vi "MainIdent RT.vi"() -> ()   [LabVIEW 2019]
doc: "The myRIO Project template acquires acceleration data from the onboard accelerometer and displays the changes of acceleration values in a waveform chart."
uses:
  CD1.ctl
  <vilib>/myRIO/Common/Instrument Driver Framework/myRIO v1.0/Encoder/typedefs/Encoder Signal Mode.ctl
  <vilib>/Platform/TimedLoop/XDataNode/timing_clust.ctl
  <vilib>/Platform/TimedLoop/XDataNode/nitl_modes.ctl
  <vilib>/Platform/TimedLoop/XDataNode/wakeup.ctl
  <vilib>/myRIO/Instrument Drivers/Onboard IO/PWM/typedefs/PWM Reference.ctl
  <vilib>/myRIO/Common/Instrument Driver Framework/Utilities/typedefs/myRIO Generic Hardware Reference.ctl
  <vilib>/myRIO/Common/Instrument Driver Framework/Utilities/typedefs/Hardware Version Enum.ctl
  <vilib>/myRIO/Common/Instrument Driver Framework/Utilities/typedefs/myRIO v1.0 Reference.ctl
  <vilib>/myRIO/Common/Instrument Driver Framework/Utilities/typedefs/Generic FPGA Reference.ctl
  <vilib>/myRIO/Common/Instrument Driver Framework/myRIO v1.0/PWM/typedefs/PWM Channels Enum.ctl
  <vilib>/myRIO/Instrument Drivers/Onboard IO/PWM/typedefs/PWM Configuration.ctl
  <vilib>/userDefined/High Color/nirio_resource_hc.ctl
  <vilib>/myRIO/Common/Instrument Driver Framework/myRIO v1.0/Encoder/typedefs/Encoder Configuration v1.0.ctl
  <vilib>/myRIO/Instrument Drivers/Onboard IO/Encoder/typedefs/Encoder Reference.ctl
  <vilib>/myRIO/Common/Instrument Driver Framework/myRIO v1.0/Encoder/typedefs/Encoder Channels Enum.ctl
  <vilib>/myRIO/Common/Instrument Driver Framework/myRIO v1.0/PWM/vis/myRIO v1.1 Open PWM.vi
  <vilib>/myRIO/Common/Instrument Driver Framework/myRIO v1.0/Encoder/vis/myRIO v1.1 Open Encoder.vi
  <vilib>/myRIO/Common/Instrument Driver Framework/Utilities/vis/Validate Channels.vi
  <vilib>/myRIO/Common/Instrument Driver Framework/myRIO v1.0/PWM/vis/myRIO v1.0 Reserve PWM.vi
  <vilib>/myRIO/Instrument Drivers/Onboard IO/PWM/vis/Set Duty Cycle and Frequency.vi
  <vilib>/myRIO/Common/Instrument Driver Framework/myRIO v1.0/Encoder/vis/myRIO v1.0 Reserve Encoder.vi
  <vilib>/myRIO/Common/Instrument Driver Framework/myRIO v1.0/Encoder/vis/myRIO v1.0 Close Encoder.vi
  <vilib>/myRIO/Common/Instrument Driver Framework/myRIO v1.0/PWM/vis/myRIO v1.0 Close PWM.vi
  <vilib>/myRIO/Common/Instrument Driver Framework/myRIO v1.0/PWM/vis/myRIO v1.0 Build MUX Configuration PWM.vi
  <vilib>/myRIO/Common/Instrument Driver Framework/myRIO v1.0/Resource Manager/vis/myRIO v1.0 Reserve Channel List.vi
  <vilib>/myRIO/Common/Instrument Driver Framework/myRIO v1.0/Encoder/vis/myRIO v1.0 Build MUX Configuration Encoder.vi
  <vilib>/myRIO/Common/Instrument Driver Framework/myRIO v1.0/Encoder/vis/myRIO v1.0 Unreserve Encoder.vi
  <vilib>/myRIO/Common/Instrument Driver Framework/myRIO v1.0/PWM/vis/myRIO v1.0 Unreserve PWM.vi
  <vilib>/myRIO/Common/Instrument Driver Framework/myRIO v1.0/Resource Manager/vis/myRIO v1.0 Create Configuration List.vi
  <vilib>/myRIO/Common/Instrument Driver Framework/myRIO v1.0/Resource Manager/vis/myRIO v1.0 Reserve Channel.vi
  <vilib>/myRIO/Common/Instrument Driver Framework/myRIO v1.0/Resource Manager/vis/myRIO v1.0 Unreserve Channel.vi
  <vilib>/myRIO/Common/Instrument Driver Framework/myRIO v1.0/Resource Manager/vis/myRIO v1.0 Unreserve Channel List.vi
  <vilib>/myRIO/Common/Instrument Driver Framework/myRIO v1.0/Resource Manager/vis/myRIO v1.0 Build Mutex Name.vi
  <vilib>/Utility/VariantDataType/GetNumericInfo.vi
  <vilib>/Utility/error.llb/Error Cluster From Error Code.vi
  <vilib>/myRIO/Common/Instrument Driver Framework/myRIO v1.0/myRIO v1.1 Open.vi
  <vilib>/myRIO/Common/Instrument Driver Framework/Utilities/vis/IO Manager.vi
  <vilib>/myRIO/Common/Instrument Driver Framework/Utilities/vis/Configuration Manager.vi
  <vilib>/myRIO/Common/Instrument Driver Framework/myRIO v1.0/Resource Manager/vis/myRIO v1.0 Configure IO.vi
  <vilib>/myRIO/Common/Instrument Driver Framework/myRIO v1.0/myRIO v1.0 Close.vi
  <vilib>/myRIO/Common/Instrument Driver Framework/myRIO v1.0/PWM/vis/myRIO v1.0 Write PWM.vi
  <vilib>/myRIO/Common/Instrument Driver Framework/myRIO v1.0/Encoder/vis/myRIO v1.0 Configure Encoder.vi
  <vilib>/myRIO/Common/Instrument Driver Framework/myRIO v1.0/Encoder/vis/myRIO v1.0 Enable Encoder.vi
  <vilib>/myRIO/Common/Instrument Driver Framework/myRIO v1.0/Encoder/vis/myRIO v1.0 Read Encoder.vi
  <vilib>/imath/engines/lvmath2/RunTimeEngine/Managers/WorkSpace/UID Generator.vi
  <vilib>/imath/engines/lvmath2/RunTimeEngine/IndexRead/NIMS V(S).vi
  <instcachedir>/0/NIMS V(S)_0488751826AF41519A22953C041130DC.lvgen/NIMS V(S)_0488751826AF41519A22953C041130DC_000.vi
  <vilib>/imath/engines/lvmath2/RunTimeEngine/BuiltInFunctions/atan2/NIMS_atan2.vi
  <instcachedir>/0/NIMS_atan2_A91AA4A7D42247EDBE8F76DB99AF04A4.lvgen/NIMS_atan2_A91AA4A7D42247EDBE8F76DB99AF04A4_000.vi
  <vilib>/imath/engines/lvmath2/RunTimeEngine/ErrorHandling/NIMS_Create Error From Enums.vi
  <vilib>/imath/engines/lvmath2/RunTimeEngine/ArithmeticOperatorToken/NIMS_ArithmeticOperator_power(S).vi
  <instcachedir>/0/NIMS_ArithmeticOperator_power(S)_F1497A2DE3CE4E82B2C3646D59904248.lvgen/NIMS_ArithmeticOperator_power(S)_F1497A2DE3CE4E82B2C3646D59904248_010.vi
  <vilib>/imath/engines/lvmath2/RunTimeEngine/BuiltInFunctions/acos/NIMS_acos(C).vi
  <instcachedir>/0/NIMS_acos(C)_835262ADAFAC4BBF9DF1C2958A624AC3.lvgen/NIMS_acos(C)_835262ADAFAC4BBF9DF1C2958A624AC3_001.vi
  <vilib>/imathl/engines/lvmath/Functions/Error Handling/Create Error.vi
  <vilib>/imath/engines/lvmath2/RunTimeEngine/RunTimeType/NIMS_RunTimeType_From StrictType (excl LVString).vi
  <instcachedir>/0/NIMS_RunTimeType_From StrictType (excl LVString)_D8AFBA86A94845AAA577C895450664BD.lvgen/NIMS_RunTimeType_From StrictType (excl LVString)_D8AFBA86A94845AAA577C895450664BD_000.vi
  <vilib>/imath/engines/lvmath2/RunTimeEngine/LocalVariableDefStatement/MC_LocalVariableDefStatement_Display.vi
  <vilib>/imath/engines/lvmath2/RunTimeEngine/RangeToken/NIMS_Range_R3 - Integer.vi
  <instcachedir>/0/NIMS_Range_R3 - Integer_E6E7B420460D4F08A65C42474AF91D7C.lvgen/NIMS_Range_R3 - Integer_E6E7B420460D4F08A65C42474AF91D7C_000.vi
  <vilib>/imath/engines/lvmath2/RunTimeEngine/CommandStatement/MC_CommandStatement_break.vi
  <vilib>/imath/engines/lvmath2/RunTimeEngine/VariableToken/NIMS_VariableToken_CondDefinedDefinedByReplace.vi
  <instcachedir>/0/NIMS_VariableToken_CondDefinedDefinedByReplace_D162CFFC24174562A9FEA619A91E1A56.lvgen/NIMS_VariableToken_CondDefinedDefinedByReplace_D162CFFC24174562A9FEA619A91E1A56_000.vi
  <vilib>/imath/engines/lvmath2/RunTimeEngine/IndexReplace/NIMS V(S)=S.vi
  <instcachedir>/0/NIMS V(S)=S_BD5C8CB81B6E4D99B8C0034EA1BEE55D.lvgen/NIMS V(S)=S_BD5C8CB81B6E4D99B8C0034EA1BEE55D_001.vi
  <vilib>/imath/engines/lvmath2/RunTimeEngine/VariableToken/NIMS_VariableToken_CondDefined.vi
  <instcachedir>/0/NIMS_VariableToken_CondDefined_30C3C94EAC01413DA882E848DEC89944.lvgen/NIMS_VariableToken_CondDefined_30C3C94EAC01413DA882E848DEC89944_000.vi
  <vilib>/imath/engines/lvmath/Functions/Error Handling/MergeErrorsWrapper.vi
  <vilib>/imath/engines/lvmath2/RunTimeEngine/Managers/SymbolTable/Clear UID.vi
  <vilib>/imath/engines/lvmath2/RunTimeEngine/NodeEndStatement/NIMS_NodeEndStatement_Output.vi
  <instcachedir>/0/NIMS_NodeEndStatement_Output_53EC0D466D134D7ABD903AC30B43404B.lvgen/NIMS_NodeEndStatement_Output_53EC0D466D134D7ABD903AC30B43404B_001.vi
  <instcachedir>/0/NIMS_NodeEndStatement_Output_53EC0D466D134D7ABD903AC30B43404B.lvgen/NIMS_NodeEndStatement_Output_53EC0D466D134D7ABD903AC30B43404B_000.vi
  <vilib>/imath/engines/lvmath2/RunTimeEngine/ErrorHandling/NIMS_Finalize Error.vi
  <instcachedir>/0/NIMS_NodeEndStatement_Output_53EC0D466D134D7ABD903AC30B43404B.lvgen/NIMS_NodeEndStatement_Output_53EC0D466D134D7ABD903AC30B43404B_009.vi
  <vilib>/myRIO/Common/Instrument Driver Framework/myRIO v1.0/Encoder/vis/myRIO v1.0 Shutdown Encoder.vi
  <vilib>/myRIO/Common/Instrument Driver Framework/myRIO v1.0/PWM/vis/myRIO v1.0 Shutdown PWM.vi
  <vilib>/platform/TimedLoop/XDataNode/XDataNode.xnode
  <vilib>/myRIO/Instrument Drivers/Onboard IO/PWM/vis/myRIO PWM Open.xnode
  <vilib>/myRIO/Instrument Drivers/Onboard IO/Encoder/vis/myRIO Encoder Open.xnode
  <vilib>/Platform/TimedLoop/XDataNode/XDNodeRunTimeDep.lvlib
  <vilib>/myRIO/Instrument Drivers/Onboard IO/Encoder/Encoder.lvlib
  <vilib>/myRIO/Instrument Drivers/Onboard IO/PWM/PWM.lvlib
  <vilib>/imath/engines/lvmath2/RunTimeEngine/Managers/SymbolTable/NIMS_WorkSpace.lvlib
panel:
  out "String 2":string
  out "data":T1
  out "String":string
  out "Numeric 16":dbl
  out "Numeric 15":dbl
  out "Numeric 14":dbl
  out "Numeric 13":dbl
  out "Numeric 12":dbl
  out "Numeric 11":dbl
  out "Numeric 10":dbl
  out "Numeric 9":dbl
  out "Numeric 8":dbl
  out "Numeric 7":dbl
  out "Numeric 6":dbl
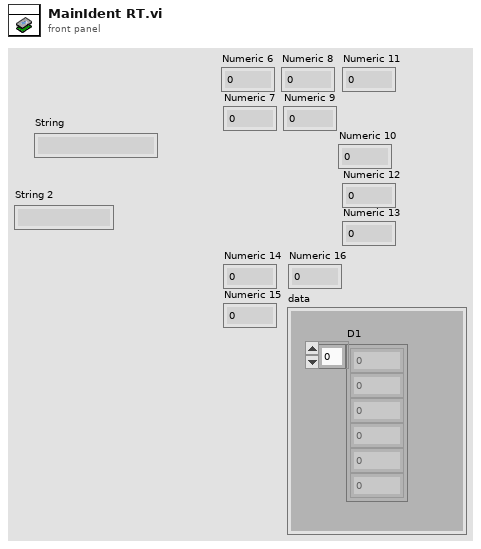
[diagram p1: front panel]
types:
  T1 = typedef "CD1.ctl" = cluster{"D1":dbl[]}
  T2 = typedef "Encoder Signal Mode.ctl" = enum16{"Quadrature phase signal", "Step and direction signal"}
  T3 = typedef "PWM.lvlib/PWM Reference.ctl" = cluster{"myRIO Reference":T4, "PWM Channels Enum":T8, "PWM Configuration":T9}
  T4 = typedef "myRIO Generic Hardware Reference.ctl" = cluster{"myRIO Model":T5, "myRIO Hardware Reference":T6}
  T5 = typedef "Hardware Version Enum.ctl" = enum16{"Unknown", "myRIO-1900", "myRIO-1950", "roboRIO", "NI ELVIS RIO CM", "ELVIS III"}
  T6 = typedef "myRIO v1.0 Reference.ctl" = cluster{"Generic FPGA Reference":T7, "Allow multiple opens":bool}
  T7 = typedef "Generic FPGA Reference.ctl" = refnum<k20>
  T8 = typedef "PWM Channels Enum.ctl" = enum16{"Not Connected", "C/PWM0", "C/PWM1", "A/PWM0", "A/PWM1", "A/PWM2", "A/PWM3", "A/PWM4", "A/PWM5", "A/PWM6", "A/PWM7", "A/PWM8", "A/PWM9", "A/PWM10", "A/PWM11", "A/PWM12", "A/PWM13", "A/PWM14", "A/PWM15", "A/PWM16", "A/PWM17", "A/PWM18", "A/PWM19", "B/PWM0", "B/PWM1", "B/PWM2", "B/PWM3", "B/PWM4", "B/PWM5", "B/PWM6", "B/PWM7", "B/PWM8", "B/PWM9", "B/PWM10", "B/PWM11", "B/PWM12", "B/PWM13", "B/PWM14", "B/PWM15", "B/PWM16", "B/PWM17", "B/PWM18", "B/PWM19", "PWM/PWM0", "PWM/PWM1", "PWM/PWM2", "PWM/PWM3", "PWM/PWM4", "PWM/PWM5", "PWM/PWM6", "PWM/PWM7", "PWM/PWM8", "PWM/PWM9"}
  T9 = typedef "PWM.lvlib/PWM Configuration.ctl" = cluster{"Frequency":dbl, "Duty Cycle":dbl}
  T10 = typedef "Encoder.lvlib/Encoder Reference.ctl" = cluster{"myRIO Reference":T4, "Encoder Channels Enum":T11}
  T11 = typedef "Encoder Channels Enum.ctl" = enum16{"Not Connected", "C/ENC0", "C/ENC1", "A/ENC", "A/ENC0", "A/ENC1", "A/ENC2", "A/ENC3", "A/ENC4", "A/ENC5", "A/ENC6", "A/ENC7", "A/ENC8", "A/ENC9", "B/ENC", "B/ENC0", "B/ENC1", "B/ENC2", "B/ENC3", "B/ENC4", "B/ENC5", "B/ENC6", "B/ENC7", "B/ENC8", "B/ENC9", "DIO/ENC0", "DIO/ENC1", "DIO/ENC2", "DIO/ENC3", "DIO/ENC4"}
  T12 = typedef "XDNodeRunTimeDep.lvlib/timing_clust.ctl" = cluster{"Expected End [f-1]":u64, "Actual End [f-1]":u64, "Finished Late? [f-1]":bool, "Expected End [i-1]":u64, "Actual End [i-1]":u64, "Finished Late? [i-1]":bool, "Expected Start [i]":u64, "Actual Start [i]":u64, "Expected Start [f]":u64, "Actual Start [f]":u64, "Source Name":string, "Structure Name":string, "Period":i64, "Deadline":i64, "Offset":i64, "Start":i64, "Priority":i32, "Timeout":i32, "Mode":T13, "Wakeup Reason":T14, "Error":errorcluster, "Source Type":string, "Secondary Source Type":string, "Global End Time":u64, "Global Start Time":u64, "Frame Duration":u64, "Iteration Duration":u64, "Assigned CPU":i32, "I/O Scan Engine Mode":u32}
  T13 = typedef "XDNodeRunTimeDep.lvlib/nitl_modes.ctl" = enum32{"No Change", "Process missed periods, maintain original phase", "Discard missed periods, maintain original phase", "Process missed periods, ignore original phase", "Discard missed periods, ignore original phase"}
  T14 = typedef "XDNodeRunTimeDep.lvlib/wakeup.ctl" = enum32{"Normal", "Aborted", "Asynchronous wakeup", "Timing source error", "Timed loop error", "Timeout"}
  T15 = cluster{dbl, dbl, dbl, "seconds since 1Jan1904":timestamp}
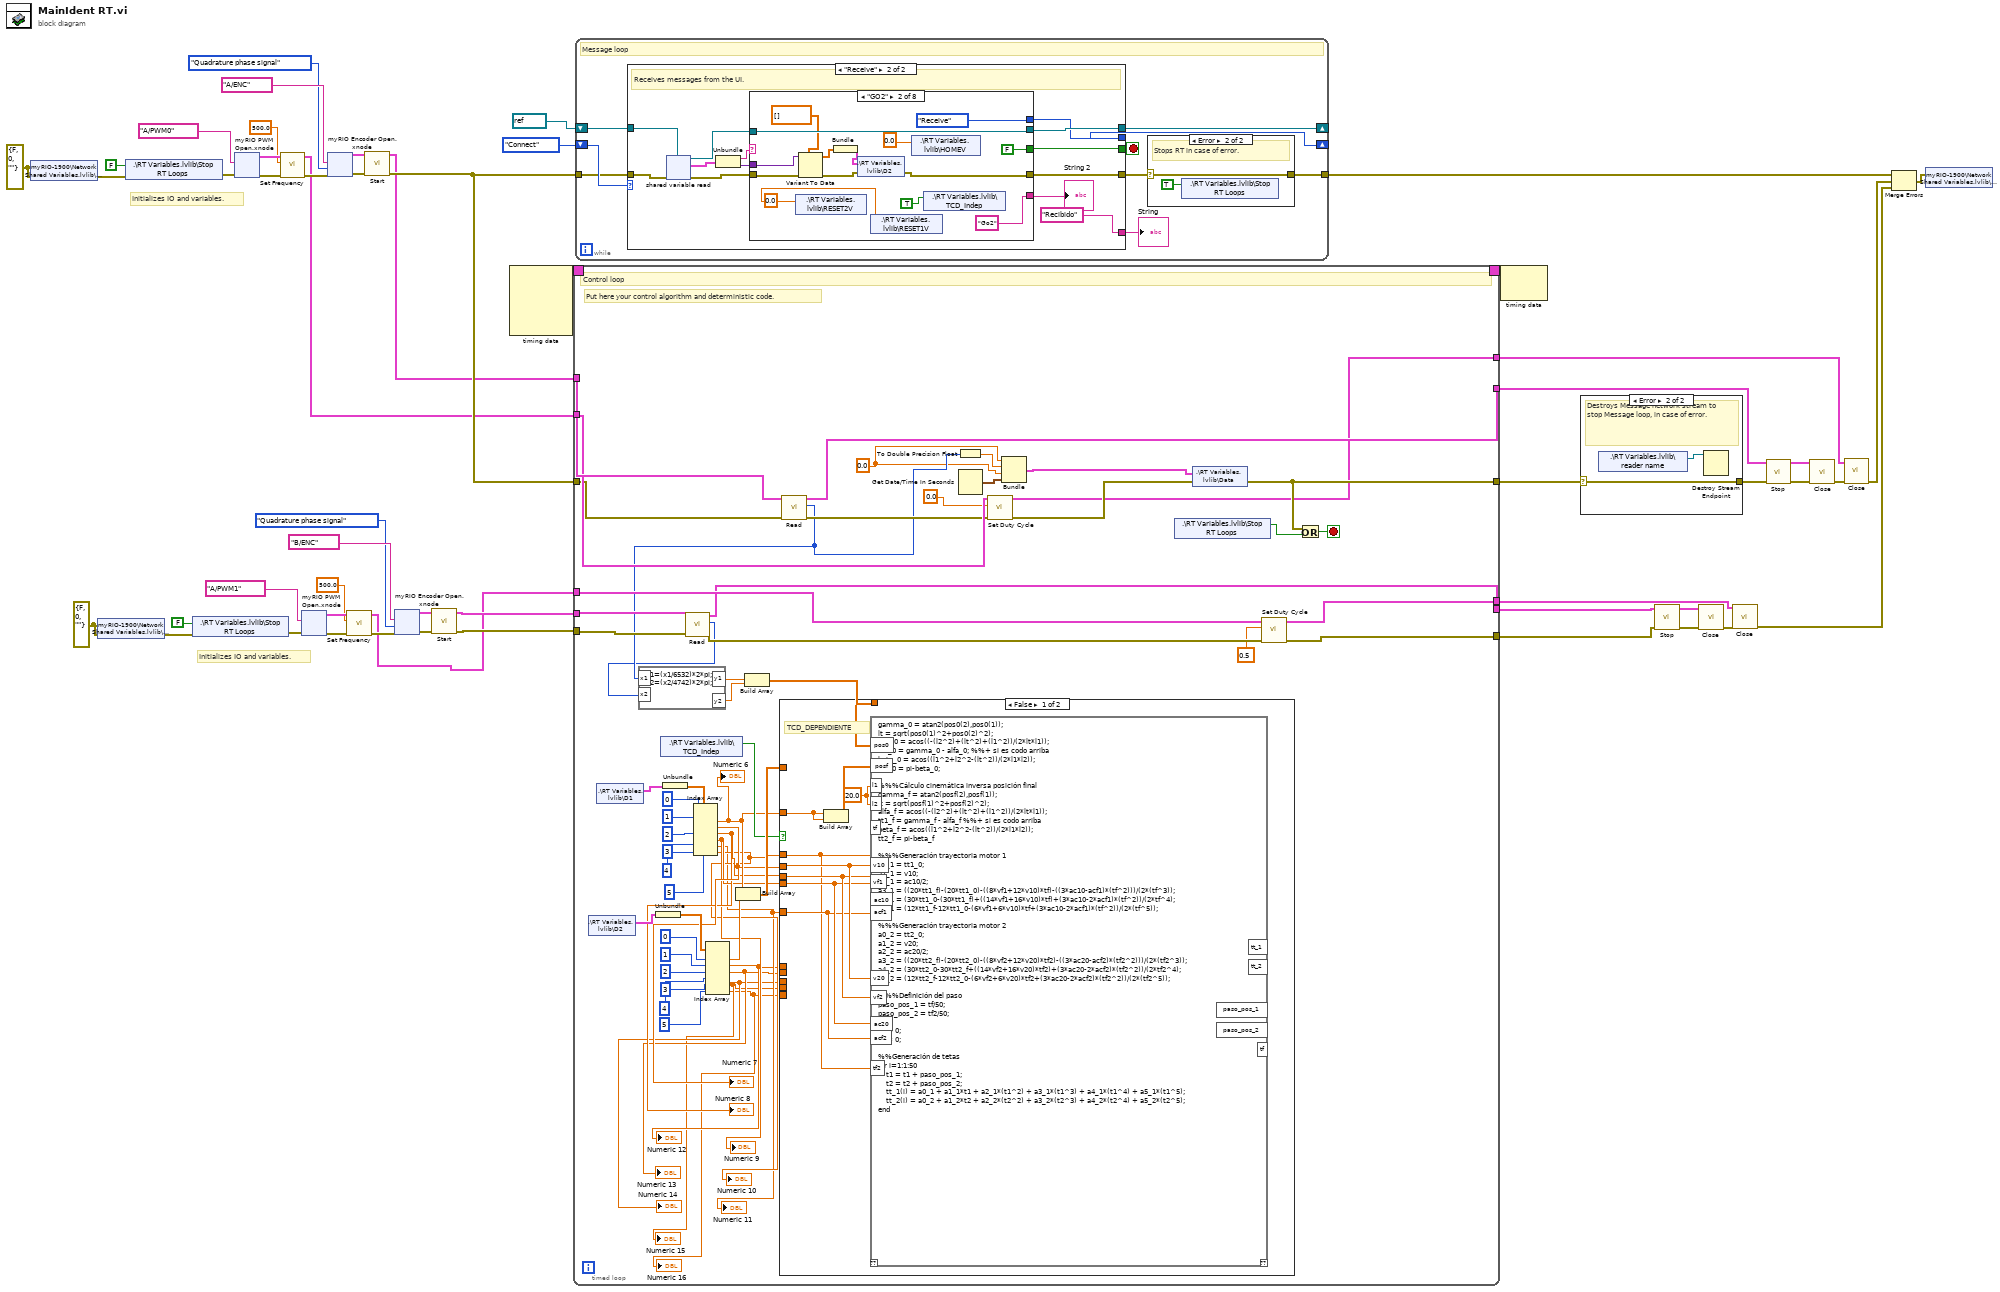
[diagram p0: block diagram]
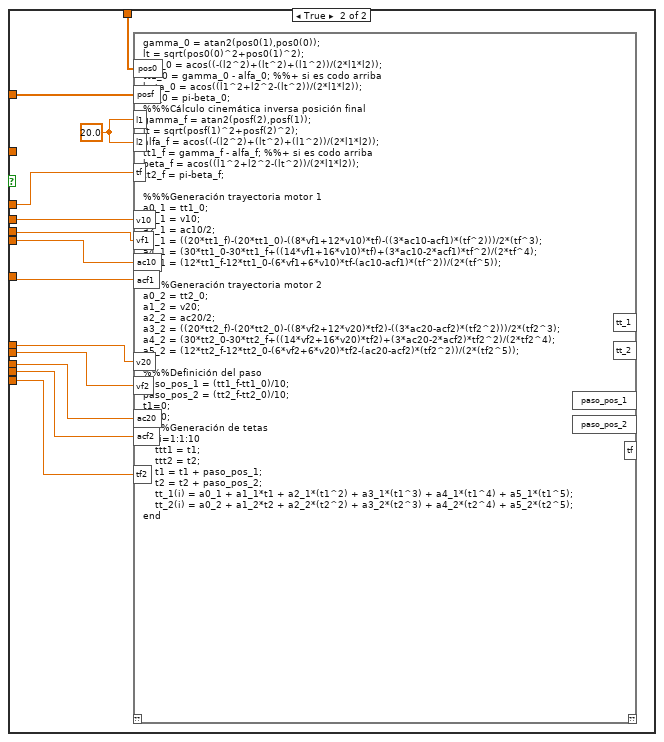
[diagram p3: hidden frame]
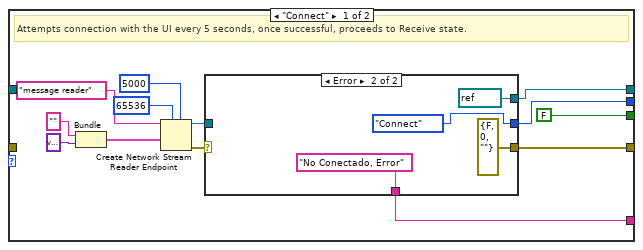
[diagram p5: hidden frame]
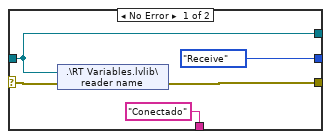
[diagram p6: hidden frame]
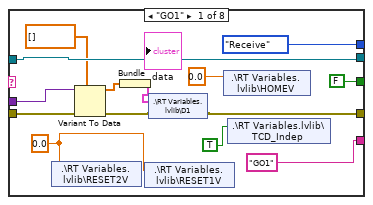
[diagram p7: hidden frame]
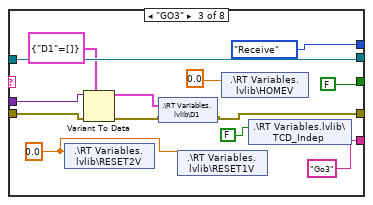
[diagram p8: hidden frame]
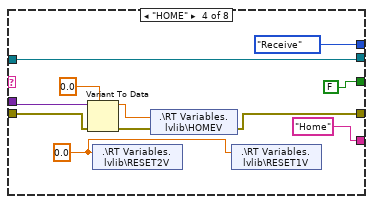
[diagram p9: hidden frame]
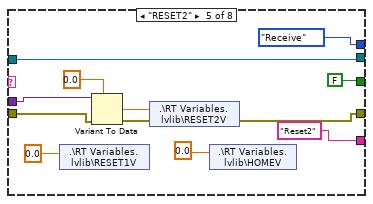
[diagram p10: hidden frame]
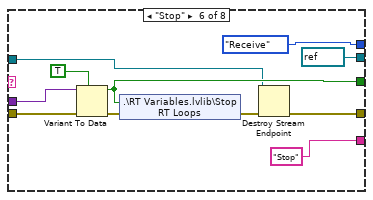
[diagram p11: hidden frame]
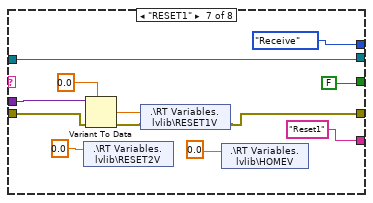
[diagram p12: hidden frame]
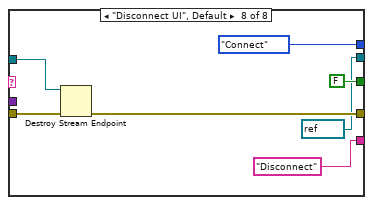
[diagram p13: hidden frame]
diagram:
  w21 = errorcluster {"status"=FALSE, "code"=0, "source"=""} ("error IO")
  w45 = errorcluster {"status"=FALSE, "code"=0, "source"=""} ("error IO")
  # "Initializes IO and variables."
  # "Initializes IO and variables."
  n1 = shared-variable "myRIO-1900\\Network Shared Variables.lvlib\\error IO"(w45, error in=w45) -> (error out=w46:errorcluster)
  n2 = shared-variable "myRIO-1900\\Network Shared Variables.lvlib\\error IO"(w21, error in=w21) -> (error out=w22:errorcluster)
  n3 = shared-variable ".\\RT Variables.lvlib\\Stop RT Loops"(FALSE ("Stop RT Loops"), error in=w46) -> (error out=w31:errorcluster)
  n4 = shared-variable ".\\RT Variables.lvlib\\Stop RT Loops"(FALSE ("Stop RT Loops"), error in=w22) -> (error out=w14:errorcluster)
  n5 = xnode "myRIO PWM Open.xnode"("error in (no error)"=w31, "Channel Name"=tag "A/PWM0") -> ("error out"=w33:errorcluster, "PWM Ref Out"=w32:T3)  [unwired: 1 in]
  n6 = call <vilib>:"Set Frequency.vi"("error in (no error)"=w33, "Frequency [Hz]"=500.0, "PWM Ref In"=w32) -> ("error out"=w30:errorcluster, "PWM Ref Out"=w27:T3)  [unwired: 6 in]
  n7 = xnode "myRIO PWM Open.xnode"("error in (no error)"=w14, "Channel Name"=tag "A/PWM1") -> ("error out"=w16:errorcluster, "PWM Ref Out"=w15:T3)  [unwired: 1 in]
  n8 = xnode "myRIO Encoder Open.xnode"("error in (no error)"=w30, "Channel Name"=tag "A/ENC", "Encoder Signal Mode"=Encoder_Signal_Mode."Quadrature phase signal") -> ("error out"=w42:errorcluster, "Encoder Ref Out"=w41:T10)  [unwired: 2 in]
  n9 = call <vilib>:"Set Frequency.vi"("error in (no error)"=w16, "Frequency [Hz]"=500.0, "PWM Ref In"=w15) -> ("error out"=w13:errorcluster, "PWM Ref Out"=w8:T3)  [unwired: 6 in]
  n10 = call <vilib>:"Start.vi"("error in (no error)"=w42, "Encoder Ref In"=w41) -> ("error out"=w39:errorcluster, "Encoder Ref Out"=w38:T10)  [unwired: 8 in]
  n11 = xnode "myRIO Encoder Open.xnode"("error in (no error)"=w13, "Channel Name"=tag "B/ENC", "Encoder Signal Mode"=Encoder_Signal_Mode."Quadrature phase signal") -> ("error out"=w19:errorcluster, "Encoder Ref Out"=w18:T10)  [unwired: 2 in]
  n12 = call <vilib>:"Start.vi"("error in (no error)"=w19, "Encoder Ref In"=w18) -> ("error out"=w9:errorcluster, "Encoder Ref Out"=w10:T10)  [unwired: 8 in]
  n13 = node-c288() -> (w53:T12)  [unwired: 4 in]
  n14 = timed-loop {
    timing: w53 -> [_]
    timing-out: [_] -> w52
    tunnel: w39 -> [w57]
    tunnel: [w108] -> w44
    tunnel: w38 -> [w107]
    tunnel: [w106] -> w34
    tunnel: w27 -> [w104]
    tunnel: [w102] -> w26
    tunnel: w10 -> [w85]
    tunnel: w9 -> [w84]
    tunnel: w8 -> [w81]
    tunnel: [w80] -> w5
    tunnel: [w79] -> w4
    tunnel: [w78] -> w2
    stop <- w109 stop-if-true
    w56 = 0.0
    # "Put here your control algorithm and deterministic code."
    # "Control loop"
    n15 = shared-variable ".\\RT Variables.lvlib\\D2"() -> (w93:T1)  [unwired: 1 in, 1 out]
    n16 = shared-variable ".\\RT Variables.lvlib\\D1"() -> (w101:T1)  [unwired: 1 in, 1 out]
    n17 = Unbundle(w93) -> ("D1"=w86:dbl[])
    n18 = shared-variable ".\\RT Variables.lvlib\\TCD_Indep"() -> (w70:bool)  [unwired: 1 in, 1 out]
    n19 = Unbundle(w101) -> ("D1"=w100:dbl[])
    n20 = call <vilib>:"Read.vi"("error in (no error)"=w84, "Encoder Ref In"=w85) -> ("error out"=w82:errorcluster, "Counter Value"=w74:i32, "Encoder Ref Out"=w78:T10)  [unwired: 5 in, 2 out]
    n21 = Index Array(array=w100, index #1=0, index #2=1, index #3=2, index #4=3, index #5=4, index #6=5) -> (element #1=w69:dbl, element #2=w68:dbl, element #3=w67:dbl, element #4=w66:dbl, element #5=w64:dbl, element #6=w65:dbl)
    "Numeric 6" <- w69
    "Numeric 7" <- w68
    "Numeric 8" <- w67
    "Numeric 9" <- w66
    "Numeric 10" <- w65
    "Numeric 11" <- w64
    n22 = Index Array(array=w86, index #1=0, index #2=1, index #3=2, index #4=3, index #5=4, index #6=5) -> (element #1=w72:dbl, element #2=w63:dbl, element #3=w62:dbl, element #4=w61:dbl, element #5=w60:dbl, element #6=w59:dbl)
    "Numeric 12" <- w63
    "Numeric 13" <- w62
    "Numeric 14" <- w61
    "Numeric 15" <- w60
    "Numeric 16" <- w59
    n23 = Build Array(w69, w72) -> (w71:dbl[])
    n24 = call <vilib>:"Read.vi"("error in (no error)"=w57, "Encoder Ref In"=w107) -> ("error out"=w83:errorcluster, "Counter Value"=w77:i32, "Encoder Ref Out"=w106:T10)  [unwired: 5 in, 2 out]
    n25 = formula code="y1=(x1/6532)*2*pi;\ny2=(x2/4742)*2*pi;"("x1"=w77, "x2"=w74) -> ("y1"=w76:dbl, "y2"=w75:dbl)
    n26 = Build Array(w76, w75) -> (w73:dbl[])
    n27 = case shown="False" w70 {
      tunnel: w73 -> [w119 w977]
      tunnel: w71 -> [_ w976]
      tunnel: w65 -> [w112 w975]
      tunnel: w59 -> [_ w974]
      tunnel: w68 -> [w116 w973]
      tunnel: w63 -> [_ w972]
      tunnel: w67 -> [w115 w971]
      tunnel: w62 -> [_ w970]
      tunnel: w66 -> [w114 w969]
      tunnel: w61 -> [_ w968]
      tunnel: w60 -> [_ w967]
      tunnel: w69 -> [w118 _]
      tunnel: w64 -> [w113 w966]
      frame False {
        w120 = 20.0
        # "TCD_DEPENDIENTE"
        n28 = Build Array(w118, w118) -> (w117:dbl[])
        n29 = mathscript code="gamma_0 = atan2(pos0(2),pos0(1));\nlt = sqrt(pos0(1)^2+pos0(2)^2);\nalfa_0 = acos((-(l2^2)+(lt^2)+(l1^2))/(2*lt*l1));\ntt1_0 = gamma_0 - alfa_0; %%+ si es codo arriba\nbeta_0 = acos((l1^2+l2^2-(lt^2))/(2*l1*l2));\ntt2_0 = pi-beta_0;\n\n%%%Cálculo cinemática inversa posición final\ngamma_f = atan2(posf(2),posf(1));\nlt = sqrt(posf(1)^2+posf(2)^2);\nalfa_f = acos((-(l2^2)+(lt^2)+(l1^2))/(2*lt*l1));\ntt1_f = gamma_f - alfa_f %%+ si es codo arriba\nbeta_f = acos((l1^2+l2^2-(lt^2))/(2*l1*l2));\ntt2_f = pi-beta_f\n\n%%%Generación trayectoria motor 1\na0_1 = tt1_0;\na1_1 = v10;\na2_1 = ac10/2;\na3_1 = ((20*tt1_f)-(20*tt1_0)-((8*vf1+12*v10)*tf)-((3*ac10-acf1)*(tf^2)))/(2*(tf^3));\na4_1 = (30*tt1_0-(30*tt1_f)+((14*vf1+16*v10)*tf)+(3*ac10-2*acf1)*(tf^2))/(2*tf^4);\na5_1 = (12*tt1_f-12*tt1_0-(6*vf1+6*v10)*tf+(3*ac10-2*acf1)*(tf^2))/(2*(tf^5));\n\n%%%Generación trayectoria motor 2\na0_2 = tt2_0;\na1_2 = v20;\na2_2 = ac20/2;\na3_2 = ((20*tt2_f)-(20*tt2_0)-((8*vf2+12*v20)*tf2)-((3*ac20-acf2)*(tf2^2)))/(2*(tf2^3));\na4_2 = (30*tt2_0-30*tt2_f+((14*vf2+16*v20)*tf2)+(3*ac20-2*acf2)*(tf2^2))/(2*tf2^4);\na5_2 = (12*tt2_f-12*tt2_0-(6*vf2+6*v20)*tf2+(3*ac20-2*acf2)*(tf2^2))/(2*(tf2^5));\n\n%%%Definición del paso\npaso_pos_1 = tf/50;\npaso_pos_2 = tf2/50;\n\nt1 = 0;\nt2 = 0;\n\n%%Generación de tetas\nfor i=1:1:50\n    t1 = t1 + paso_pos_1;\n    t2 = t2 + paso_pos_2;\n    tt_1(i) = a0_1 + a1_1*t1 + a2_1*(t1^2) + a3_1*(t1^3) + a4_1*(t1^4) + a5_1*(t1^5);\n    tt_2(i) = a0_2 + a1_2*t2 + a2_2*(t2^2) + a3_2*(t2^3) + a4_2*(t2^4) + a5_2*(t2^5);\nend"("pos0"=w119, "posf"=w117, "l1"=w120, "l2"=w120, "tf"=w112, "v10"=w116, "vf1"=w115, "ac10"=w114, "acf1"=w113, "tf2"=w112, "v20"=w116, "ac20"=w114, "vf2"=w115, "acf2"=w113) -> ()  [unwired: 1 in, 6 out]
      }
      frame True {
        w978 = 20.0
        n30 = mathscript code="gamma_0 = atan2(pos0(1),pos0(0));\nlt = sqrt(pos0(0)^2+pos0(1)^2);\nalfa_0 = acos((-(l2^2)+(lt^2)+(l1^2))/(2*l1*l2));\ntt1_0 = gamma_0 - alfa_0; %%+ si es codo arriba\nbeta_0 = acos((l1^2+l2^2-(lt^2))/(2*l1*l2));\ntt2_0 = pi-beta_0;\n%%%Cálculo cinemática inversa posición final\ngamma_f = atan2(posf(2),posf(1));\nlt = sqrt(posf(1)^2+posf(2)^2);\nalfa_f = acos((-(l2^2)+(lt^2)+(l1^2))/(2*l1*l2));\ntt1_f = gamma_f - alfa_f; %%+ si es codo arriba\nbeta_f = acos((l1^2+l2^2-(lt^2))/(2*l1*l2));\ntt2_f = pi-beta_f;\n\n%%%Generación trayectoria motor 1\na0_1 = tt1_0;\na1_1 = v10;\na2_1 = ac10/2;\na3_1 = ((20*tt1_f)-(20*tt1_0)-((8*vf1+12*v10)*tf)-((3*ac10-acf1)*(tf^2)))/2*(tf^3);\na4_1 = (30*tt1_0-30*tt1_f+((14*vf1+16*v10)*tf)+(3*ac10-2*acf1)*tf^2)/(2*tf^4);\na5_1 = (12*tt1_f-12*tt1_0-(6*vf1+6*v10)*tf-(ac10-acf1)*(tf^2))/(2*(tf^5));\n\n%%%Generación trayectoria motor 2\na0_2 = tt2_0;\na1_2 = v20;\na2_2 = ac20/2;\na3_2 = ((20*tt2_f)-(20*tt2_0)-((8*vf2+12*v20)*tf2)-((3*ac20-acf2)*(tf2^2)))/2*(tf2^3);\na4_2 = (30*tt2_0-30*tt2_f+((14*vf2+16*v20)*tf2)+(3*ac20-2*acf2)*tf2^2)/(2*tf2^4);\na5_2 = (12*tt2_f-12*tt2_0-(6*vf2+6*v20)*tf2-(ac20-acf2)*(tf2^2))/(2*(tf2^5));\n\n%%%Definición del paso\npaso_pos_1 = (tt1_f-tt1_0)/10;\npaso_pos_2 = (tt2_f-tt2_0)/10;\nt1=0;\nt2=0;\n%%%Generación de tetas\nfor i=1:1:10\n    ttt1 = t1;\n    ttt2 = t2;\n    t1 = t1 + paso_pos_1;\n    t2 = t2 + paso_pos_2;\n    tt_1(i) = a0_1 + a1_1*t1 + a2_1*(t1^2) + a3_1*(t1^3) + a4_1*(t1^4) + a5_1*(t1^5);\n    tt_2(i) = a0_2 + a1_2*t2 + a2_2*(t2^2) + a3_2*(t2^3) + a4_2*(t2^4) + a5_2*(t2^5);    \nend"("pos0"=w977, "posf"=w976, "l1"=w978, "l2"=w978, "tf"=w975, "v10"=w973, "vf1"=w971, "ac10"=w969, "acf1"=w966, "tf2"=w974, "v20"=w972, "ac20"=w968, "vf2"=w970, "acf2"=w967) -> ()  [unwired: 1 in, 6 out]
      }
    }
    n31 = To Double Precision Float(number=w77) -> (double precision float=w103:dbl)
    n32 = Get Date/Time In Seconds() -> (seconds since 1Jan1904=w111:timestamp)
    n33 = call <vilib>:"Set Duty Cycle.vi"("error in (no error)"=w83, "Duty Cycle"=0.0, "PWM Ref In"=w104) -> ("error out"=w105:errorcluster, "PWM Ref Out"=w102:T3)  [unwired: 6 in]
    n34 = Bundle(w56, w103, w56, "seconds since 1Jan1904"=w111) -> (w54:T15)  [unwired: 1 in]
    n35 = shared-variable ".\\RT Variables.lvlib\\Stop RT Loops"() -> (w110:bool)  [unwired: 1 in, 1 out]
    n36 = shared-variable ".\\RT Variables.lvlib\\Data"(w54, error in=w105) -> (error out=w108:errorcluster)
    n37 = call <vilib>:"Set Duty Cycle.vi"("error in (no error)"=w82, "Duty Cycle"=0.5, "PWM Ref In"=w81) -> ("error out"=w80:errorcluster, "PWM Ref Out"=w79:T3)  [unwired: 6 in]
    n38 = Or(x=w108, y=w110) -> (x .or. y?=w109:bool)
  }
  n39 = while {
    tunnel: [w1846] -> w48
    shift-right: [w1852] -> _
    shift-left: refnum<k21> refnum ("reader name") -> [w1850]
    shift-right: [w1851] -> _
    shift-left: enum16{"Connect", "Receive"}."Connect" ("Message states") -> [w1853]
    tunnel: w39 -> [w1848]
    stop <- w1849 stop-if-true
    # "Message loop"
    n40 = case shown="\"Receive\"" w1853 {
      tunnel: [w1860 w1884] -> w1847
      tunnel: [w1859 w1886] -> w1852
      tunnel: [w1867 w1881] -> w1851
      tunnel: w1850 -> [_ w1891]
      tunnel: w1848 -> [_ w1883]
      tunnel: [FALSE ("Stop RT Loops") w1882] -> w1849
      tunnel: [w1857 "Recibido"] -> w1845
      frame "Connect" {
        # "Attempts connection with the UI every 5 seconds, once successful, proceeds to Receive state."
        n41 = Bundle("", variant) -> (w1863:cluster{string, variant})  [unwired: 1 in]
        n42 = Create Network Stream Reader Endpoint(5:5000 ("timeout in ms (-1)"), 7:65536 ("reader buffer size"), 9:w1863, 11:"message reader" ("reader name")) -> (0:w1862:errorcluster, 3:w1858:refnum<k21>)  [unwired: 3 in]
        n43 = case shown="Error" w1862 {
          selector: w1862 -> [w1872 _]
          tunnel: [enum16{"Connect", "Receive"}."Receive" ("Message states") enum16{"Connect", "Receive"}."Connect" ("Message states")] -> w1867
          tunnel: [w1871 errorcluster {"status"=FALSE, "code"=0, "source"=""} ("error IO")] -> w1860
          tunnel: [w1873 refnum<k21> refnum ("reader name")] -> w1859
          tunnel: w1858 -> [w1873 _]
          tunnel: ["Conectado" "No Conectado, Error"] -> w1857
          frame No Error {
            n44 = shared-variable ".\\RT Variables.lvlib\\reader name"(w1873, error in=w1872) -> (error out=w1871:errorcluster)
          }
          frame Error {
          }
        }
      }
      frame "Receive" {
        # "Receives messages from the UI."
        n45 = shared-variable-read(w1891, w1883) -> (w1885:refnum<k21>, w1887:errorcluster, w1890:cluster{string, variant})  [unwired: 1 in, 1 out]
        n46 = Unbundle(w1890) -> (w1889:string, w1888:variant)
        n47 = case shown="\"GO2\"" w1889 {
          tunnel: w1888 -> [w1905 w1917 w1929 w1938 w1951 w1964 w1974 _]
          tunnel: w1887 -> [w1904 w1918 w1928 w1939 w1950 w1966 w1975 w1983]
          tunnel: [w1899 w1913 w1925 w1935 w1947 w1960 w1970 w1982] -> w1884
          tunnel: [w1903 w1919 w1932 w1943 w1955 refnum<k21> refnum ("reader name") w1978 refnum<k21> refnum ("reader name")] -> w1886
          tunnel: w1885 -> [w1903 w1919 w1932 w1943 w1955 w1959 w1978 w1981]
          tunnel: [FALSE ("Stop RT Loops") FALSE ("Stop RT Loops") FALSE ("Stop RT Loops") FALSE ("Stop RT Loops") FALSE ("Stop RT Loops") w1963 FALSE ("Stop RT Loops") FALSE ("Stop RT Loops")] -> w1882
          tunnel: [enum16{"Connect", "Receive"}."Receive" ("Message states") enum16{"Connect", "Receive"}."Receive" ("Message states") enum16{"Connect", "Receive"}."Receive" ("Message states") enum16{"Connect", "Receive"}."Receive" ("Message states") enum16{"Connect", "Receive"}."Receive" ("Message states") enum16{"Connect", "Receive"}."Receive" ("Message states") enum16{"Connect", "Receive"}."Receive" ("Message states") enum16{"Connect", "Receive"}."Connect" ("Message states")] -> w1881
          tunnel: ["GO1" "Go2" "Go3" "Home" "Reset2" "Stop" "Reset1" "Disconnect"] -> w1879
          frame "GO1" {
            w1897 = 0.0
            n48 = shared-variable ".\\RT Variables.lvlib\\RESET2V"(w1897) -> ()  [unwired: 1 in, 1 out]
            n49 = Variant To Data(error in=w1904, type=dbl[] [] ("appended array"), Variant=w1905) -> (data=w1893:dbl[], error out=w1900:errorcluster)
            n50 = Bundle("appended array"=w1893) -> (w1892:cluster{"appended array":dbl[]})  [unwired: 1 in]
            n51 = shared-variable ".\\RT Variables.lvlib\\RESET1V"(w1897) -> ()  [unwired: 1 in, 1 out]
            n52 = shared-variable ".\\RT Variables.lvlib\\D1"(w1892, error in=w1900) -> (error out=w1899:errorcluster)
            n53 = shared-variable ".\\RT Variables.lvlib\\HOMEV"(0.0) -> ()  [unwired: 1 in, 1 out]
            n54 = shared-variable ".\\RT Variables.lvlib\\TCD_Indep"(TRUE) -> ()  [unwired: 1 in, 1 out]
          }
          frame "GO2" {
            w1911 = 0.0
            n55 = shared-variable ".\\RT Variables.lvlib\\RESET2V"(w1911) -> ()  [unwired: 1 in, 1 out]
            n56 = Variant To Data(error in=w1918, type=dbl[] [] ("appended array"), Variant=w1917) -> (data=w1907:dbl[], error out=w1914:errorcluster)
            n57 = Bundle("appended array"=w1907) -> (w1906:cluster{"appended array":dbl[]})  [unwired: 1 in]
            n58 = shared-variable ".\\RT Variables.lvlib\\D2"(w1906, error in=w1914) -> (error out=w1913:errorcluster)
            n59 = shared-variable ".\\RT Variables.lvlib\\RESET1V"(w1911) -> ()  [unwired: 1 in, 1 out]
            n60 = shared-variable ".\\RT Variables.lvlib\\HOMEV"(0.0) -> ()  [unwired: 1 in, 1 out]
            n61 = shared-variable ".\\RT Variables.lvlib\\TCD_Indep"(TRUE) -> ()  [unwired: 1 in, 1 out]
          }
          frame "GO3" {
            w1922 = 0.0
            n62 = shared-variable ".\\RT Variables.lvlib\\RESET2V"(w1922) -> ()  [unwired: 1 in, 1 out]
            n63 = Variant To Data(error in=w1928, type=T1 {"D1"=[]} ("D1"), Variant=w1929) -> (data=w1924:T1, error out=w1926:errorcluster)
            n64 = shared-variable ".\\RT Variables.lvlib\\D1"(w1924, error in=w1926) -> (error out=w1925:errorcluster)
            n65 = shared-variable ".\\RT Variables.lvlib\\RESET1V"(w1922) -> ()  [unwired: 1 in, 1 out]
            n66 = shared-variable ".\\RT Variables.lvlib\\HOMEV"(0.0) -> ()  [unwired: 1 in, 1 out]
            n67 = shared-variable ".\\RT Variables.lvlib\\TCD_Indep"(FALSE) -> ()  [unwired: 1 in, 1 out]
          }
          frame "HOME" {
            w1934 = 0.0
            n68 = Variant To Data(error in=w1939, type=0.0, Variant=w1938) -> (data=w1937:dbl, error out=w1936:errorcluster)
            n69 = shared-variable ".\\RT Variables.lvlib\\RESET2V"(w1934) -> ()  [unwired: 1 in, 1 out]
            n70 = shared-variable ".\\RT Variables.lvlib\\HOMEV"(w1937, error in=w1936) -> (error out=w1935:errorcluster)
            n71 = shared-variable ".\\RT Variables.lvlib\\RESET1V"(w1934) -> ()  [unwired: 1 in, 1 out]
          }
          frame "RESET2" {
            n72 = shared-variable ".\\RT Variables.lvlib\\RESET1V"(0.0) -> ()  [unwired: 1 in, 1 out]
            n73 = Variant To Data(error in=w1950, type=0.0, Variant=w1951) -> (data=w1948:dbl, error out=w1949:errorcluster)
            n74 = shared-variable ".\\RT Variables.lvlib\\RESET2V"(w1948, error in=w1949) -> (error out=w1947:errorcluster)
            n75 = shared-variable ".\\RT Variables.lvlib\\HOMEV"(0.0) -> ()  [unwired: 1 in, 1 out]
          }
          frame "Stop" {
            n76 = Variant To Data(error in=w1966, type=TRUE ("Stop RT Loops"), Variant=w1964) -> (data=w1963:bool, error out=w1965:errorcluster)
            n77 = shared-variable ".\\RT Variables.lvlib\\Stop RT Loops"(w1963, error in=w1965) -> (error out=w1961:errorcluster)
            n78 = Destroy Stream Endpoint(8:w1961, 11:w1959) -> (0:w1960:errorcluster)
          }
          frame "RESET1" {
            n79 = shared-variable ".\\RT Variables.lvlib\\RESET2V"(0.0) -> ()  [unwired: 1 in, 1 out]
            n80 = Variant To Data(error in=w1975, type=0.0, Variant=w1974) -> (data=w1972:dbl, error out=w1971:errorcluster)
            n81 = shared-variable ".\\RT Variables.lvlib\\RESET1V"(w1972, error in=w1971) -> (error out=w1970:errorcluster)
            n82 = shared-variable ".\\RT Variables.lvlib\\HOMEV"(0.0) -> ()  [unwired: 1 in, 1 out]
          }
          frame "Disconnect UI", Default {
            n83 = Destroy Stream Endpoint(8:w1983, 11:w1981) -> (0:w1982:errorcluster)
          }
        }
        "String 2" <- w1879
      }
    }
    "String" <- w1845
    n84 = case shown="Error" w1847 {
      selector: w1847 -> [w1854 w1855]
      tunnel: [w1854 w1855] -> w1846
      frame No Error {
        # "No action required."
      }
      frame Error {
        # "Stops RT in case of error."
        n85 = shared-variable ".\\RT Variables.lvlib\\Stop RT Loops"(TRUE ("Stop RT Loops")) -> ()  [unwired: 1 in, 1 out]
      }
    }
  }
  n86 = node-c288(w52) -> ()  [unwired: 1 out]
  n87 = case shown="Error" w44 {
    selector: w44 -> [w1986 w1987]
    tunnel: [w1986 w1987] -> w35
    frame No Error {
      # "No action required."
    }
    frame Error {
      # "Destroys Message network stream to stop Message loop, in case of error."
      n88 = shared-variable ".\\RT Variables.lvlib\\reader name"() -> (w1988:refnum<k21>)  [unwired: 1 in, 1 out]
      n89 = Destroy Stream Endpoint(11:w1988) -> ()  [unwired: 1 in, 1 out]
    }
  }
  n90 = call <vilib>:"Stop.vi"("error in (no error)"=w5, "Encoder Ref In"=w2) -> ("error out"=w7:errorcluster, "Encoder Ref Out"=w3:T10)  [unwired: 8 in]
  n91 = call <vilib>:"Close.vi"("error in (no error)"=w7, "Encoder Ref In"=w3) -> ("error out"=w6:errorcluster)  [unwired: 9 in]
  n92 = call <vilib>:"Close.vi"("error in (no error)"=w6, "PWM Ref In"=w4) -> ("error out"=w1:errorcluster)  [unwired: 9 in]
  n93 = call <vilib>:"Stop.vi"("error in (no error)"=w35, "Encoder Ref In"=w34) -> ("error out"=w36:errorcluster, "Encoder Ref Out"=w37:T10)  [unwired: 8 in]
  n94 = call <vilib>:"Close.vi"("error in (no error)"=w36, "Encoder Ref In"=w37) -> ("error out"=w29:errorcluster)  [unwired: 9 in]
  n95 = call <vilib>:"Close.vi"("error in (no error)"=w29, "PWM Ref In"=w26) -> ("error out"=w28:errorcluster)  [unwired: 9 in]
  n96 = Merge Errors(w48, w28, w1) -> (w47:errorcluster)
  n97 = shared-variable "myRIO-1900\\Network Shared Variables.lvlib\\error IO"(w47) -> ()  [unwired: 1 in, 1 out]
